vi "COM.vi"(8 "error in (no error)":errorcluster, 10 "Command":string, 11 "VISA Refnum in":refnum<visa-resource-name>="COM3") -> (0 "error out":errorcluster, 2 "Response":string="\r\n", 3 "VISA Refnum out":refnum<visa-resource-name>)   [LabVIEW 2019, in "KH7008.lvlib"]
uses:
  KH7008.lvlib
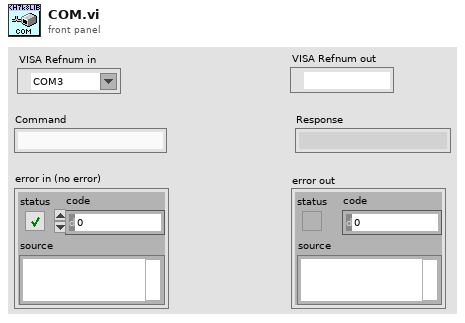
[diagram p1: front panel]
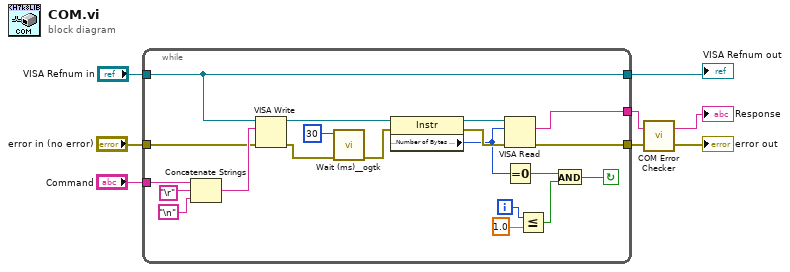
[diagram p0: block diagram]
diagram:
  n1 = while {
    tunnel: "VISA Refnum in" -> [w12]
    tunnel: "Command" -> [w22]
    tunnel: "error in (no error)" -> [w16]
    tunnel: [w23] -> w5
    tunnel: [w15] -> w2
    tunnel: [w12] -> w1
    i -> [w20]
    stop <- w17 continue-if-true
    n2 = Concatenate Strings(w22, "\r", "\n") -> (w28:string)
    n3 = VISA Write(VISA resource name=w12, write buffer=w28, error in (no error)=w16) -> (VISA resource name out=w25:refnum<visa-resource-name>, error out=w24:errorcluster)  [unwired: 1 out]
    n4 = call <userlib>:"Wait (ms)__ogtk.vi"("error in (no error)"=w24, "milliseconds to wait"=u32 30) -> ("error out"=w13:errorcluster)  [unwired: 8 in, 1 out]
    n5 = property class="Instr"(reference=w25, error in=w13) -> (reference out=w26:refnum<visa-resource-name>, error out=w10:errorcluster, "Serial Settings:Number of Bytes at Serial Port"=w9:u32)
    n6 = VISA Read(VISA resource name=w26, byte count=w9, error in (no error)=w10) -> (read buffer=w15:string, error out=w23:errorcluster)  [unwired: 2 out]
    n7 = Equal To 0?(x=w9) -> (x = 0?=w19:bool)
    n8 = Less Or Equal?(x=w20, y=1.0) -> (x <= y?=w18:bool)
    n9 = And(x=w19, y=w18) -> (x .and. y?=w17:bool)
  }
  "VISA Refnum out" <- w1
  n10 = call "COM Error Checker.vi"("error in (no error)"=w5, "String In"=w2) -> ("error out"=→"error out":errorcluster, "String"=→"Response":string)
